vi "CuLab_Exp_Avg_SGL.vi"(7 "exp Avg Factor":sgl, 8 "error in (no error)":errorcluster, 11 "T1D_SGL in":refnum<class "T1D_SGL.lvclass">) -> (0 "error out":errorcluster, 3 "T1D_SGL out":refnum<class "T1D_SGL.lvclass">)   [LabVIEW 2020]
uses:
  <vilib>/Ngene/CuLab - GPU Accelerated Toolkit/Toolkit/Low_Level/Tensor_Classes/T_Children/T1D/T1D_Children/T1D_SGL/T1D_SGL.lvclass
  C:/Program Files/National Instruments/LabVIEW 2020/vi.lib/Ngene/CuLab - GPU Accelerated Toolkit/Toolkit/Low_Level/Tensor_Classes/T_Children/T1D/T1D.lvclass
  C:/Program Files/National Instruments/LabVIEW 2020/vi.lib/Ngene/CuLab - GPU Accelerated Toolkit/Toolkit/Low_Level/Tensor_Classes/Tensor.lvclass
  0b5c155d-a4d6-4980-ab6d-1b8c98c1a38e.vi
  <vilib>/Ngene/CuLab - GPU Accelerated Toolkit/Toolkit/API/Array/Array Size/CU_Array_Size_T1D.vi
  <vilib>/Ngene/CuLab - GPU Accelerated Toolkit/Toolkit/API/Numeric/Multiply/T1D/CU_MultiplyC_T1D_SGL.vi
  <vilib>/Ngene/CuLab - GPU Accelerated Toolkit/Toolkit/Low_Level/Tensor_Classes/T_Children/T1D/T1D_Children/T1D_SGL/Set.vi
  <vilib>/Ngene/CuLab - GPU Accelerated Toolkit/Toolkit/API/Numeric/Add/T1D/CU_Add_T1D_SGL.vi
  <vilib>/Ngene/CuLab - GPU Accelerated Toolkit/Toolkit/CuLab.lvlib
  C:/Program Files/National Instruments/LabVIEW 2020/vi.lib/Ngene/CuLab - GPU Accelerated Toolkit/Toolkit/Low_Level/Tensor_Classes/T_Children/T1D/T1D_Children/T1D_SGL/T1D_SGL.lvclass
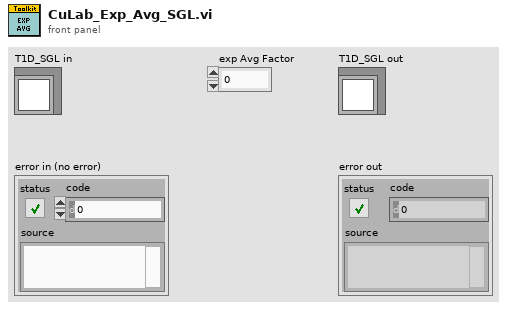
[diagram p1: front panel]
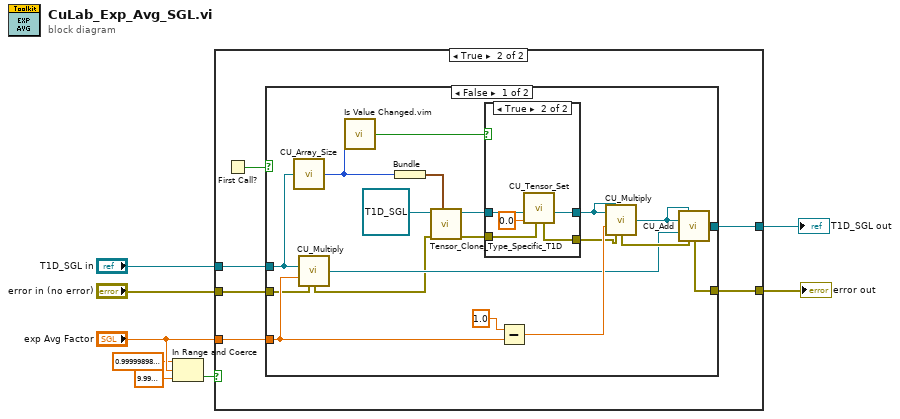
[diagram p0: block diagram]
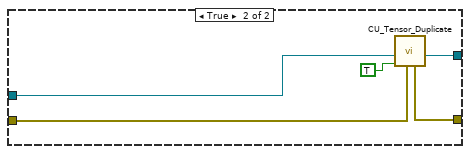
[diagram p4: hidden frame]
diagram:
  n1 = In Range and Coerce(upper limit=sgl 0.999999, x="exp Avg Factor", lower limit=sgl 1e-06) -> (In Range?=w4:bool)  [unwired: 1 out]
  n2 = case shown="True" w4 {
    tunnel: "exp Avg Factor" -> [_ w16]
    tunnel: [w9 w15] -> w8
    tunnel: [w10 w14] -> w7
    tunnel: "T1D_SGL in" -> [w9 w12]
    tunnel: "error in (no error)" -> [w10 w11]
    frame False {
    }
    frame True {
      n3 = First Call?() -> (First Call?: T/F=w13:bool)
      n4 = case shown="False" w13 {
        tunnel: [w32 w47] -> w14
        tunnel: [w31 w45] -> w15
        tunnel: w16 -> [w30 _]
        tunnel: w12 -> [w28 w43]
        tunnel: w11 -> [w29 w44]
        frame False {
          n5 = call-poly <vilib>:"CU_Array_Size.vi"("Tensor"=w28) -> ("size"=w25:i32)  [unwired: 14 in]
          n6 = call-poly <vilib>:"CU_Multiply.vi"("x"=w28, "y"=w30, "error in (no error)"=w29) -> ("Dest out"=w27:refnum<class "T1D_SGL.lvclass">, "error out"=w19:errorcluster)  [unwired: 11 in]
          n7 = call "Is Value Changed.vim"("value"=w25) -> ("changed or first call?"=w20:bool)
          n8 = Bundle("size"=w25) -> (w22:cluster{"size":i32})  [unwired: 1 in]
          n9 = call <vilib>:"Tensor_Clone_Type_Specific_T1D.vi"("Dest_Tensor_Dims"=w22, "error in (no error)"=w19, "Dest_Tensor"=refnum<class "T1D_SGL.lvclass"> refnum ("Dest out")) -> ("error out"=w18:errorcluster, "Dest_Tensor out"=w23:refnum<class "T1D_SGL.lvclass">)  [unwired: 7 in]
          n10 = case shown="True" w20 {
            tunnel: [w37 w42] -> w24
            tunnel: w23 -> [w37 w41]
            tunnel: w18 -> [w36 w39]
            tunnel: [w36 w38] -> w17
            frame False {
            }
            frame True {
              n11 = call-poly <vilib>:"CU_Tensor_Set.vi"("error in (no error)"=w39, "Value"=sgl 0.0, "T1D_SGL in"=w41) -> ("T1D_SGL out"=w42:refnum<class "T1D_SGL.lvclass">, "error out"=w38:errorcluster)  [unwired: 7 in]
            }
          }
          n12 = Subtract(x=sgl 1.0 ("y"), y=w30) -> (x-y=w34:sgl)
          n13 = call-poly <vilib>:"CU_Multiply.vi"("Dest in"=w24, "x"=w24, "y"=w34, "error in (no error)"=w17) -> ("Dest out"=w26:refnum<class "T1D_SGL.lvclass">, "error out"=w33:errorcluster)  [unwired: 10 in]
          n14 = call-poly <vilib>:"CU_Add.vi"("Dest in"=w26, "x"=w26, "y"=w27, "error in (no error)"=w33) -> ("Dest out"=w31:refnum<class "T1D_SGL.lvclass">, "error out"=w32:errorcluster)  [unwired: 10 in]
        }
        frame True {
          n15 = call <vilib>:"CU_Tensor_Duplicate.vi"("error in (no error)"=w44, "Copy Data?"=TRUE, "Tensor in"=w43) -> ("Duplicate out"=w45:refnum<class "T1D_SGL.lvclass">, "error out"=w47:errorcluster)  [unwired: 7 in]
        }
      }
    }
  }
  "T1D_SGL out" <- w8
  "error out" <- w7
